vi "Operator Input click on choice.vi"(8 "error in (no error)":errorcluster, 9 "button2 text":string, 10 "button1 text":string, 11 "Operator text":string) -> (0 "error out":errorcluster, 2 "button2 clicked?":bool, 3 "button1 clicked?":bool)   [LabVIEW 2024]
panel:
  in  "button2 clicked":bool caption="button2 clicked?"
  in  "button1 clicked":bool caption="button1 clicked?"
  out "Message":string
  # "Operator Message"
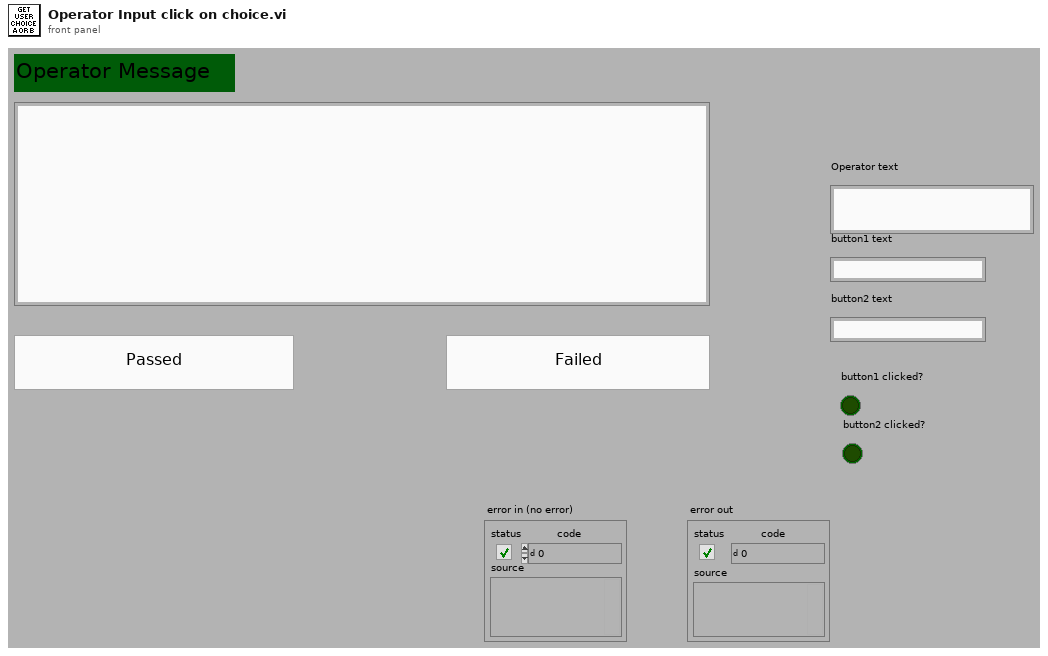
[diagram p1: front panel]
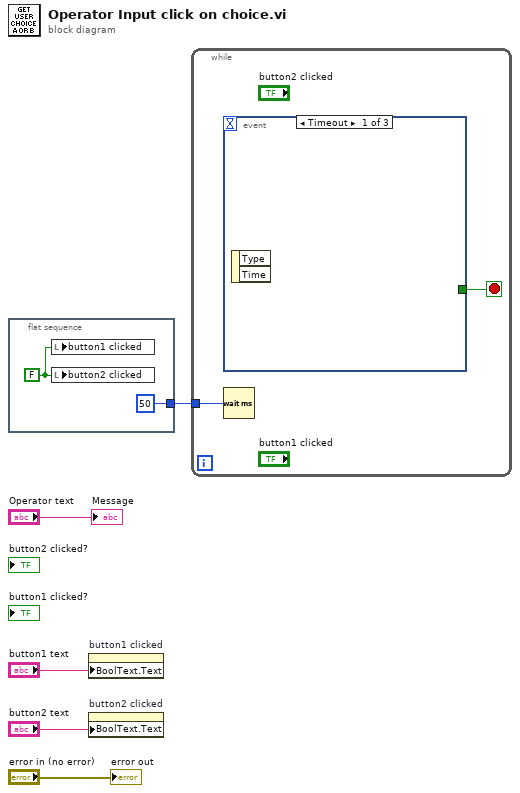
[diagram p0: block diagram]
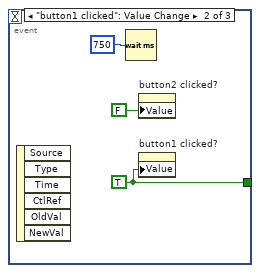
[diagram p2: hidden frame]
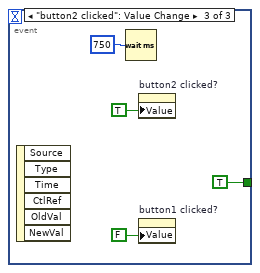
[diagram p3: hidden frame]
diagram:
  n1 = flat-sequence {
    tunnel: [u32 50 ("milliseconds to wait")] -> w5
    frame #0 {
      w6 = FALSE ("button1")
      n2 = local write "button1 clicked"(w6) -> ()
      n3 = local write "button2 clicked"(w6) -> ()
    }
  }
  n4 = property on="button1 clicked" class="Bool (strict)"("BoolText.Text"="button1 text") -> ()  [unwired: 2 in, 2 out]
  n5 = property on="button2 clicked" class="Bool (strict)"("BoolText.Text"="button2 text") -> ()  [unwired: 2 in, 2 out]
  n6 = while {
    tunnel: w5 -> [w9]
    stop <- w8 stop-if-true
    n7 = event shown="[0] Timeout" {
      selector: _ -> [_ _ _]
      dyn-events: _ -> [_ _ _]
      timeout: _ -> [_ _ _]
      tunnel: [_ w12 TRUE] -> w8
      event Timeout {
        n8 = event-data() -> ()  [unwired: 1 in, 2 out]
      }
      event "button1 clicked": Value Change {
        w12 = TRUE
        n9 = event-data() -> ()  [unwired: 1 in, 6 out]
        n10 = Wait (ms)(milliseconds to wait=u32 750) -> ()  [unwired: 1 out]
        n11 = property on="button2 clicked?" class="Bool (strict)"("Value"=FALSE ("button2 clicked?")) -> ()  [unwired: 2 in, 2 out]
        n12 = property on="button1 clicked?" class="Bool (strict)"("Value"=w12) -> ()  [unwired: 2 in, 2 out]
      }
      event "button2 clicked": Value Change {
        n13 = event-data() -> ()  [unwired: 1 in, 6 out]
        n14 = Wait (ms)(milliseconds to wait=u32 750) -> ()  [unwired: 1 out]
        n15 = property on="button2 clicked?" class="Bool (strict)"("Value"=TRUE ("button2 clicked?")) -> ()  [unwired: 2 in, 2 out]
        n16 = property on="button1 clicked?" class="Bool (strict)"("Value"=FALSE ("button1 clicked?")) -> ()  [unwired: 2 in, 2 out]
      }
    }
    n17 = Wait (ms)(milliseconds to wait=w9) -> ()  [unwired: 1 out]
  }
  "Message" <- "Operator text"
  "error out" <- "error in (no error)"
